vi "Camera Example.vi"() -> ()   [LabVIEW 2012]
doc: "Example VI: Displays an image from one of Baxter's cameras"
uses:
  <userlib>/ROS for LabVIEW Software/ROS/Code/SubVIs/BaxterCamera.ctl
panel:
  in  "stop":bool
  out "image":picture
  out "Cameras List":T1={"Number of Cameras"=3, "Cameras"=["head_camera", "left_hand_camera", "right_hand_camera"], "OK Byte"=0}
  in  "Camera Settings":T3={"Camera"=enum."left_hand_camera", "FPS"=20.0, "Camera Controls"=[], "Resolution"=enum."(320, 200)"}
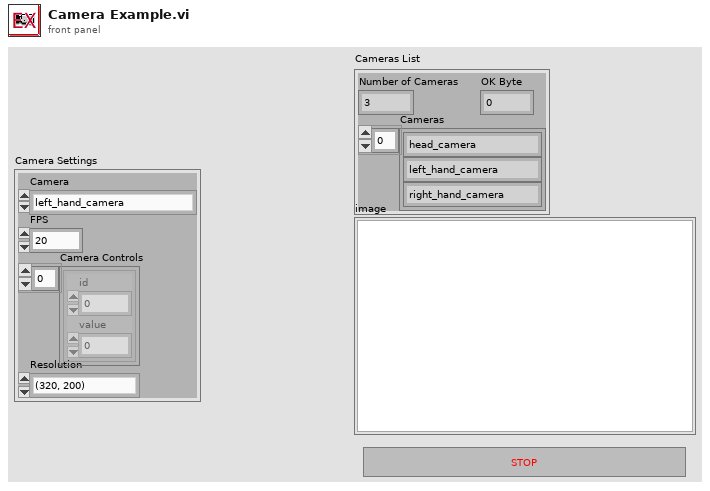
[diagram p1: front panel]
types:
  T1 = cluster{"Number of Cameras":i32, "Cameras":string[], "OK Byte":u8}
  T2 = typedef "BaxterCamera.ctl" = enum16{"left_hand_camera", "right_hand_camera", "head_camera"}
  T3 = cluster{"Camera":T2, "FPS":sgl, "Camera Controls":cluster{"id":i32, "value":i32}[], "Resolution":enum16{"(1280, 800)", "(960, 600)", "(640, 400)", "(480, 300)", "(384, 240)", "(320, 200)"}}
  T4 = typedef "imagedata.ctl" = cluster{"image type":i32, "image depth":i32, "image":u8[], "mask":u8[], "colors":u32[], "Rectangle":cluster{"left":i16, "top":i16, "right":i16, "bottom":i16}}
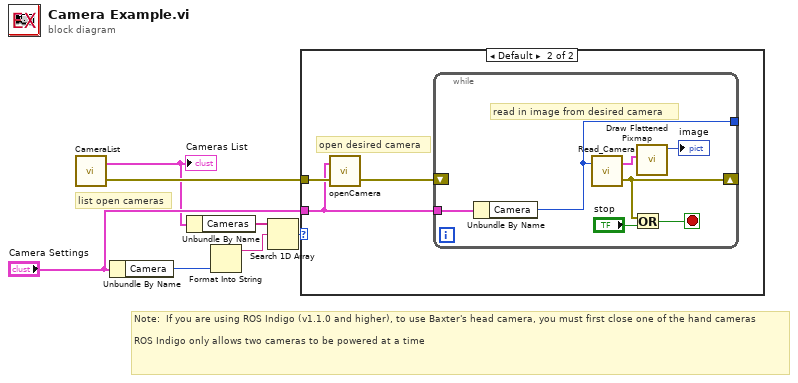
[diagram p0: block diagram]
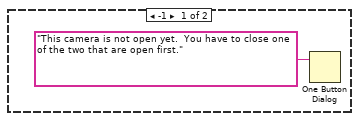
[diagram p2: hidden frame]
diagram:
  # "Note:  If you are using ROS Indigo (v1.1.0 and higher), to use Baxter's head camera, you must first close one of the hand cameras\n\nROS Indigo only allows two cameras to be powered at a time"
  # "list open cameras"
  n1 = call <userlib>:"CameraList.vi"() -> ("error out"=w7:errorcluster, "Cameras List"=w5:T1)  [unwired: 2 in]
  "Cameras List" <- w5
  n2 = Unbundle By Name("Camera Settings") -> ("Camera"=w4:T2)
  n3 = Unbundle By Name(w5) -> ("Cameras"=w3:string[])
  n4 = Format Into String(w4) -> (resulting string=w2:string)  [unwired: 3 in, 1 out]
  n5 = Search 1D Array(1D array=w3, element=w2) -> (index of element=w1:i32)  [unwired: 1 in]
  n6 = case shown="Default" w1 {
    tunnel: w7 -> [_ w11]
    tunnel: "Camera Settings" -> [_ w9]
    frame -1 {
      n7 = One Button Dialog(message="This camera is not open yet.  You have to close one of the two that are open first.") -> ()  [unwired: 1 in, 1 out]
    }
    frame Default {
      # "open desired camera"
      n8 = call <userlib>:"openCamera.vi"("error in"=w11, "Camera Settings"=w9) -> ("error out"=w10:errorcluster)  [unwired: 2 in]
      n9 = while {
        tunnel: w9 -> [w16]
        shift-right: [w14] -> _
        shift-left: w10 -> [_]
        tunnel: [w12] -> _
        stop <- w13 stop-if-true
        # "read in image from desired camera"
        n10 = Unbundle By Name(w16) -> ("Camera"=w12:T2)
        n11 = call <userlib>:"Read_Camera.vi"("Camera"=w12) -> ("error out"=w14:errorcluster, "image data"=w18:T4)  [unwired: 2 in]
        n12 = Or(x=w14, y="stop") -> (x .or. y?=w13:bool)
        n13 = call <vilib>:"Draw Flattened Pixmap.vi"("image data"=w18) -> ("new picture"=→"image":picture)  [unwired: 8 in]
      }
    }
  }
